vi "Set Database.vi"(8 "error in (no error)":errorcluster, 10 "Database":refnum<class "Database Interface.lvclass">, 11 "Basic Column Configuration in":refnum<class "Column Configuration.lvclass">) -> (0 "error out":errorcluster, 3 "Basic Column Configuration out":refnum<class "Column Configuration.lvclass">)   [LabVIEW 2020, in "Column Interfaces.lvlib" / "Column Configuration.lvclass"]
uses:
  Column Configuration.lvclass
  Database Libraries/Database Interfaces/Database Interface Class/Database Interface.lvclass
  Column Configuration.lvclass/Column Configuration.ctl
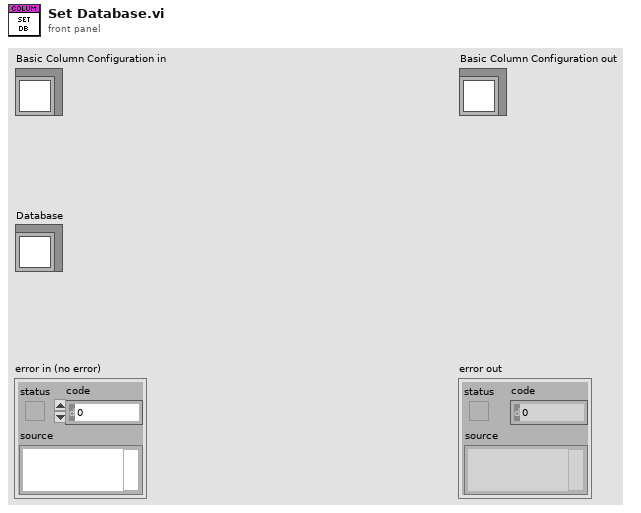
[diagram p1: front panel]
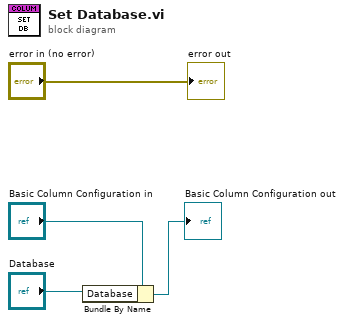
[diagram p0: block diagram]
diagram:
  n1 = Bundle By Name(cluster="Basic Column Configuration in", "Database"="Database") -> (→"Basic Column Configuration out":refnum<class "Column Configuration.lvclass">)
  "error out" <- "error in (no error)"
